vi "PSA Acquire Zspan.vi"(8 "error in (no error)":errorcluster, 9 "Sweep Time (s)":dbl=0.02, 10 "Center Frequency (Hz)":dbl=1000000000.0, 11 "VISA Refnum in":refnum<visa-resource-name>) -> (0 "error out":errorcluster, 2 "captured waveform":waveform(dbl)(graph), 3 "VISA Refnum out":refnum<visa-resource-name>)   [LabVIEW 2014]
uses:
  Agilent ESA PSA Series/Configure Frequency (Center Span).vi
  Agilent ESA PSA Series.lvlib
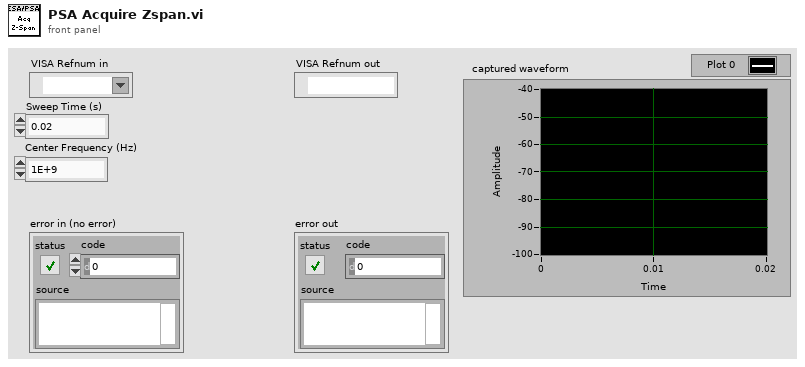
[diagram p1: front panel]
types:
  T1 = cluster{"Initial X":dbl, "X Increment":dbl, "Trace Array":dbl[]}
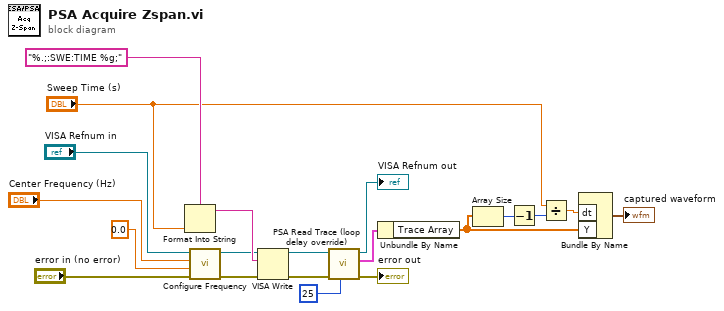
[diagram p0: block diagram]
diagram:
  n1 = Format Into String(format string="%.;:SWE:TIME %g;", "Sweep Time (s)") -> (resulting string=w19:string)  [unwired: 2 in, 1 out]
  n2 = call-poly "Configure Frequency.vi"("error in (no error)"="error in (no error)", "Span (2 GHz)"=0.0 ("Span (2.65E+10 Hz)"), "Center Frequency (2 GHz)"="Center Frequency (Hz)", "VISA resource name"="VISA Refnum in") -> ("error out"=w15:errorcluster, "VISA resource name out"=w13:refnum<visa-resource-name>)  [unwired: 6 in]
  n3 = VISA Write(VISA resource name=w13, write buffer=w19, error in (no error)=w15) -> (VISA resource name out=w12:refnum<visa-resource-name>, error out=w10:errorcluster)  [unwired: 1 out]
  n4 = call "PSA Read Trace (loop delay override).vi"("loop delay (ms)"=u32 25, "error in (no error)"=w10, "VISA resource name"=w12) -> ("error out"=→"error out":errorcluster, "Trace Waveform"=w9:T1, "VISA resource name out"=→"VISA Refnum out":refnum<visa-resource-name>)  [unwired: 6 in]
  n5 = Unbundle By Name(w9) -> ("Trace Array"=w4:dbl[])
  n6 = Array Size(array=w4) -> (size(s)=w2:i32)
  n7 = Decrement(x=w2) -> (x-1=w1:i32)
  n8 = Divide(x="Sweep Time (s)", y=w1) -> (x/y=w3:dbl)
  n9 = Bundle By Name("dt"=w3, "Y"=w4) -> (→"captured waveform":waveform(dbl))  [unwired: 1 in]
